vi "iTCread.vi"(0 "VISA resource name":refnum<visa-resource-name>, 1 "iTCreadCtrl":T1, 3 "error in (no error)":errorcluster) -> (7 "VISA resource name out":refnum<visa-resource-name>, 8 "number":dbl, 9 "read buffer":string, 10 "error out":errorcluster)   [LabVIEW 2017]
uses:
  controls/iTCreadCtrl.ctl
  <vilib>/regexp/Match Regular Expression.xnode
panel:
  out "read buffer 2":string
  out "after match":string
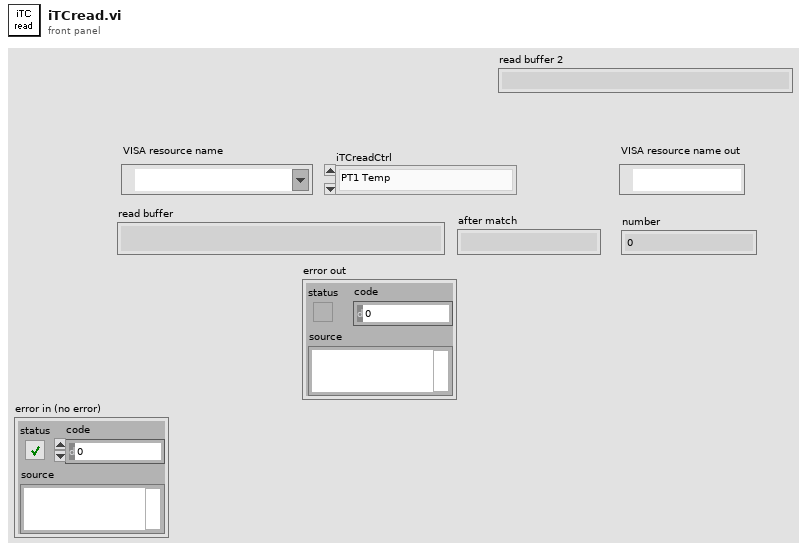
[diagram p1: front panel]
types:
  T1 = typedef "iTCreadCtrl.ctl" = enum16{"PT1 Temp", "PT2 Temp", "Sample Temp", "VTI Temp", "Needle Valve", "VTI Heater Power", "Sample Heater Power", "VTI Pressure"}
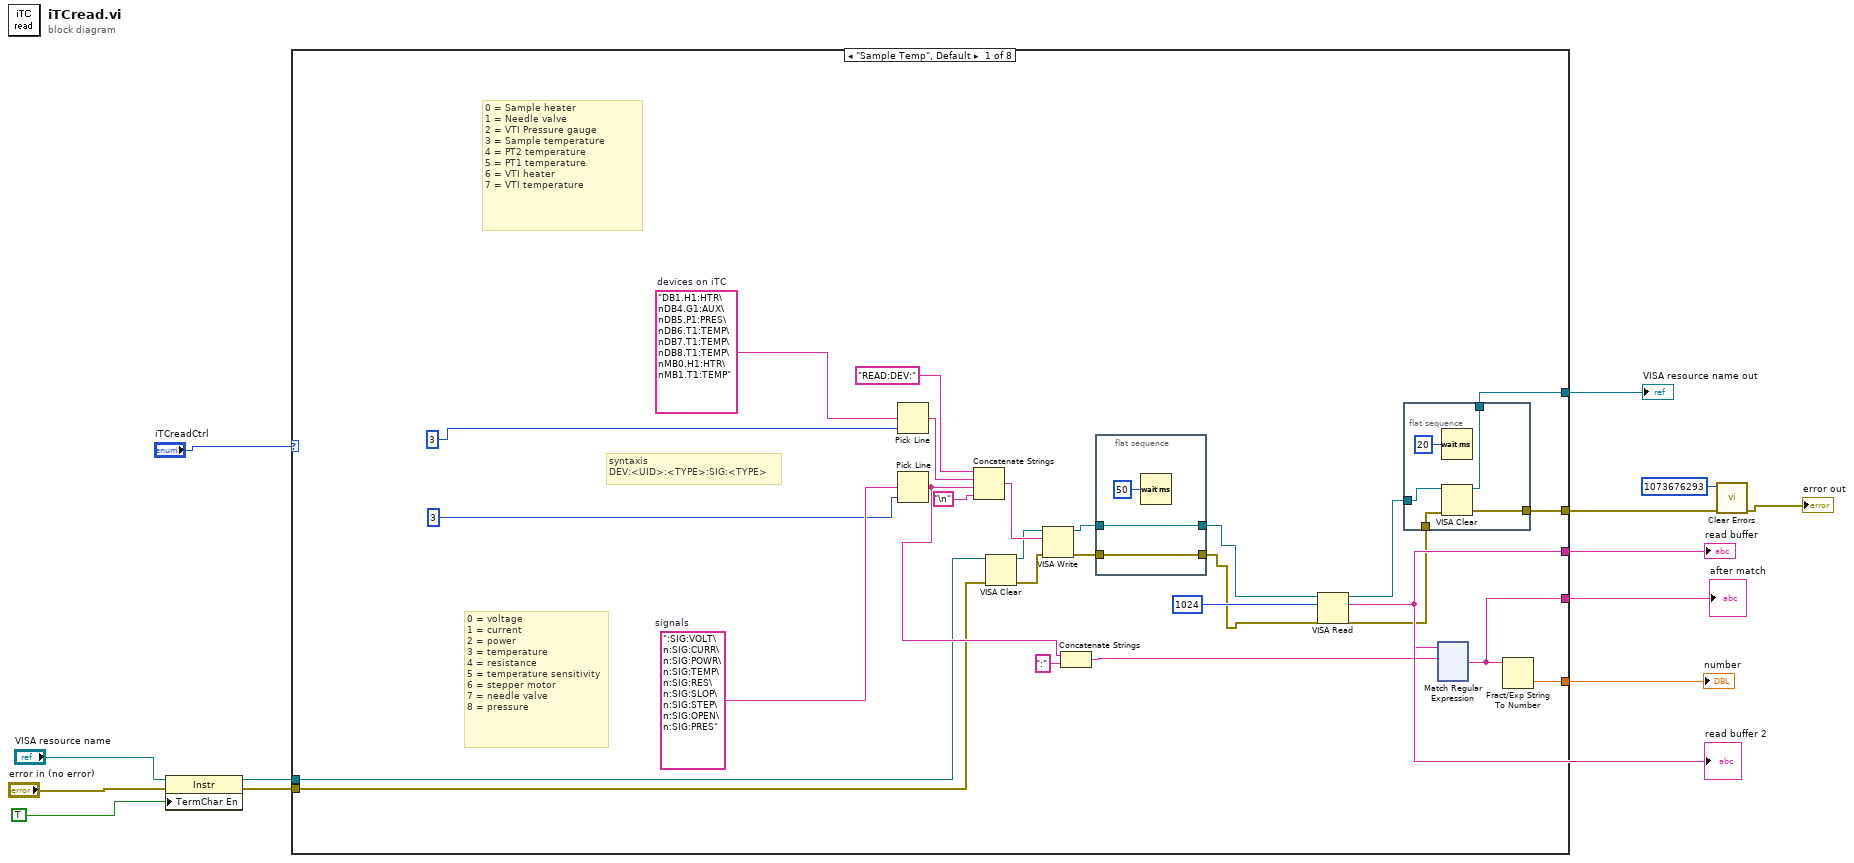
[diagram p0: block diagram]
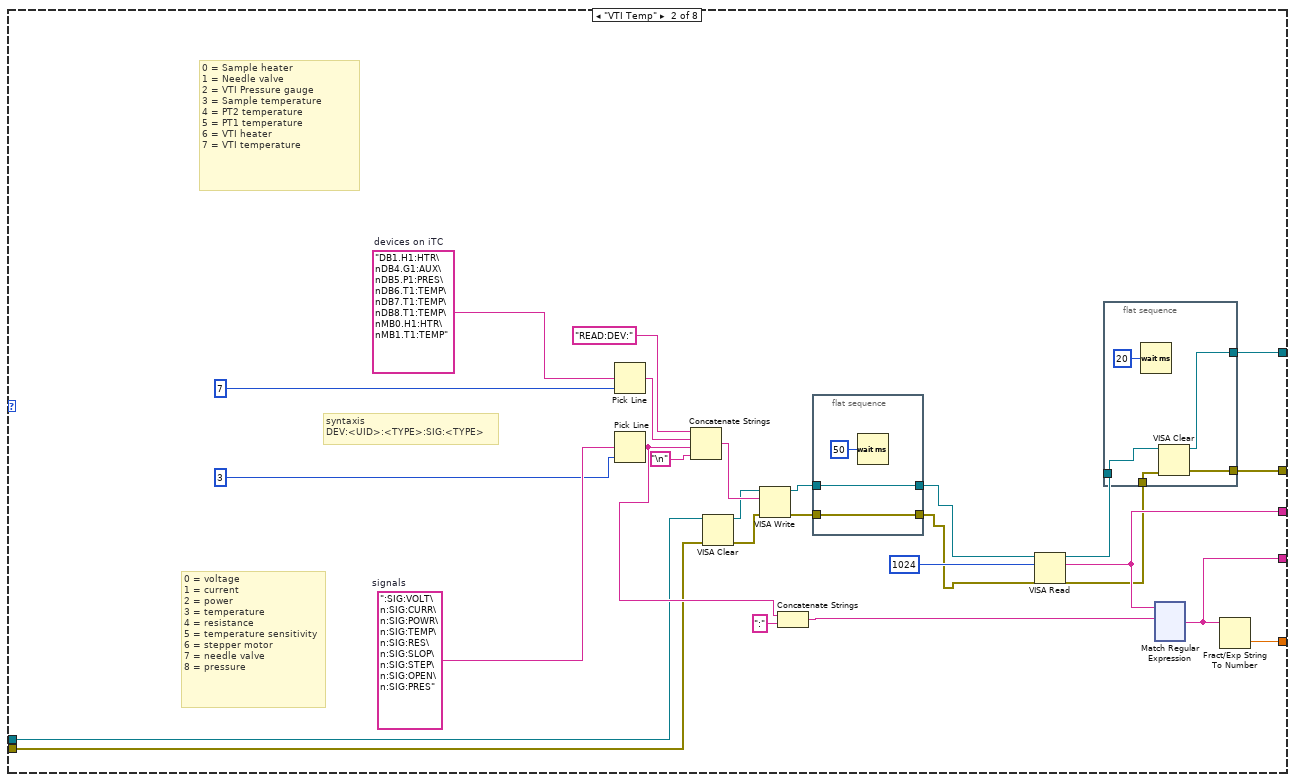
[diagram p2: hidden frame]
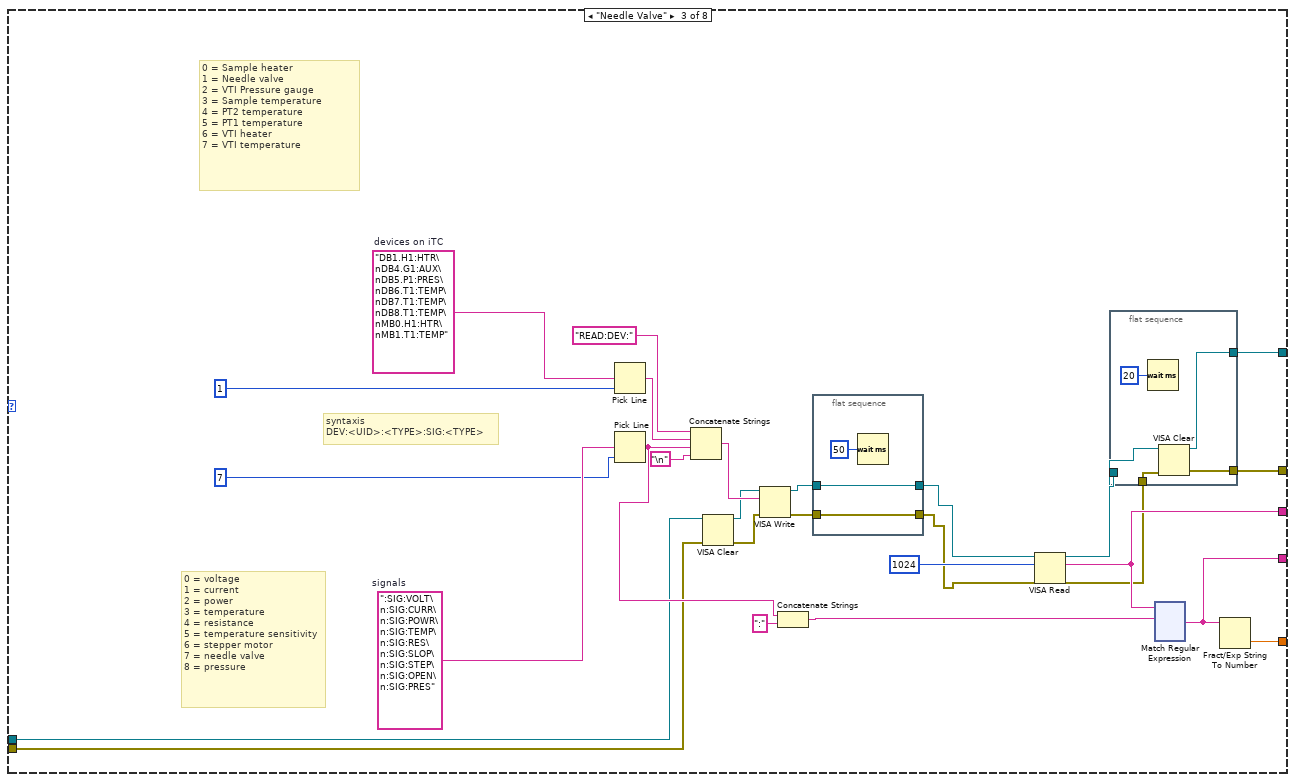
[diagram p3: hidden frame]
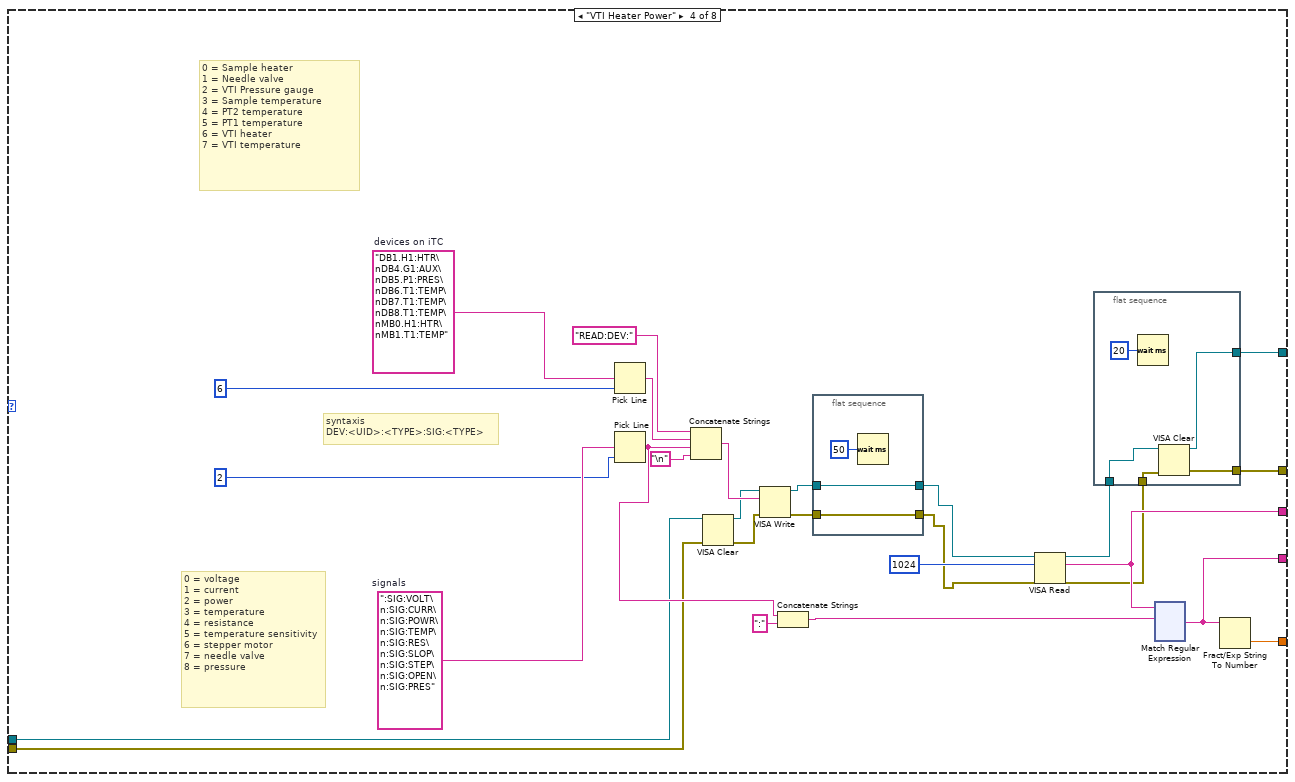
[diagram p4: hidden frame]
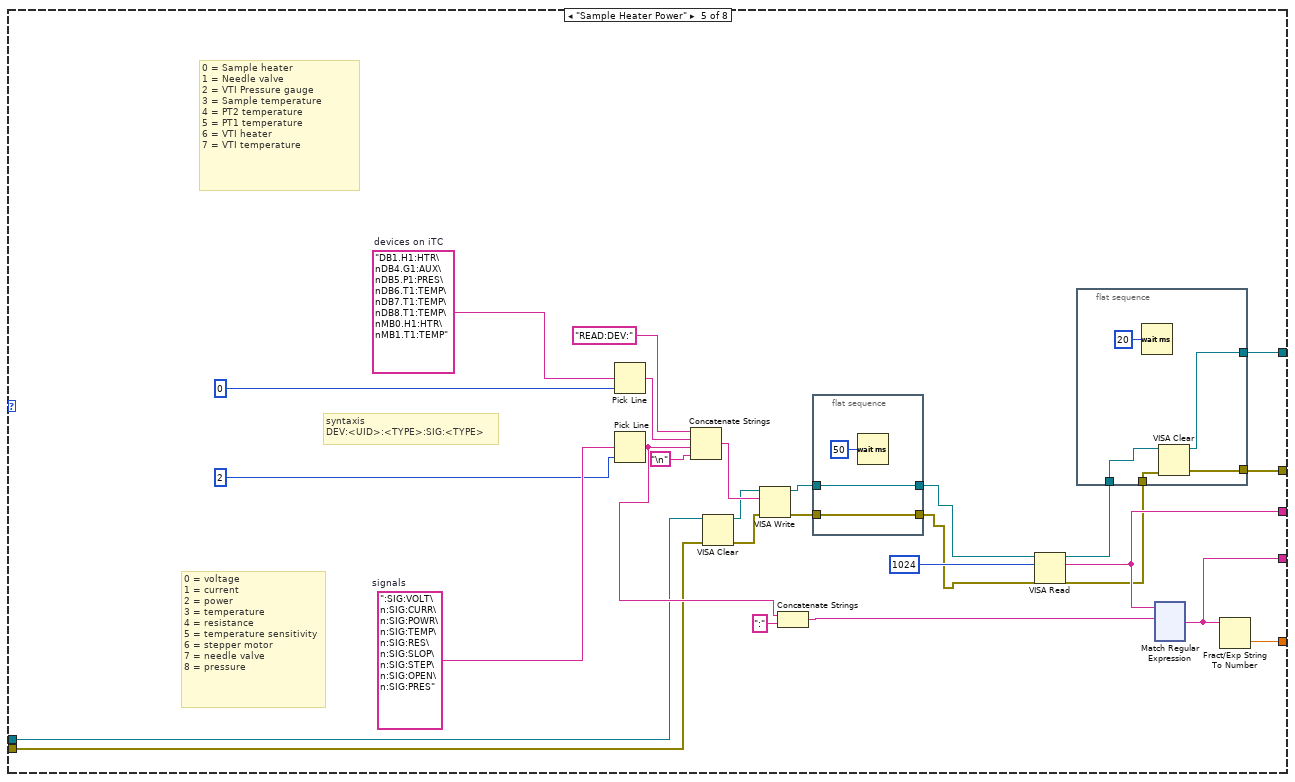
[diagram p5: hidden frame]
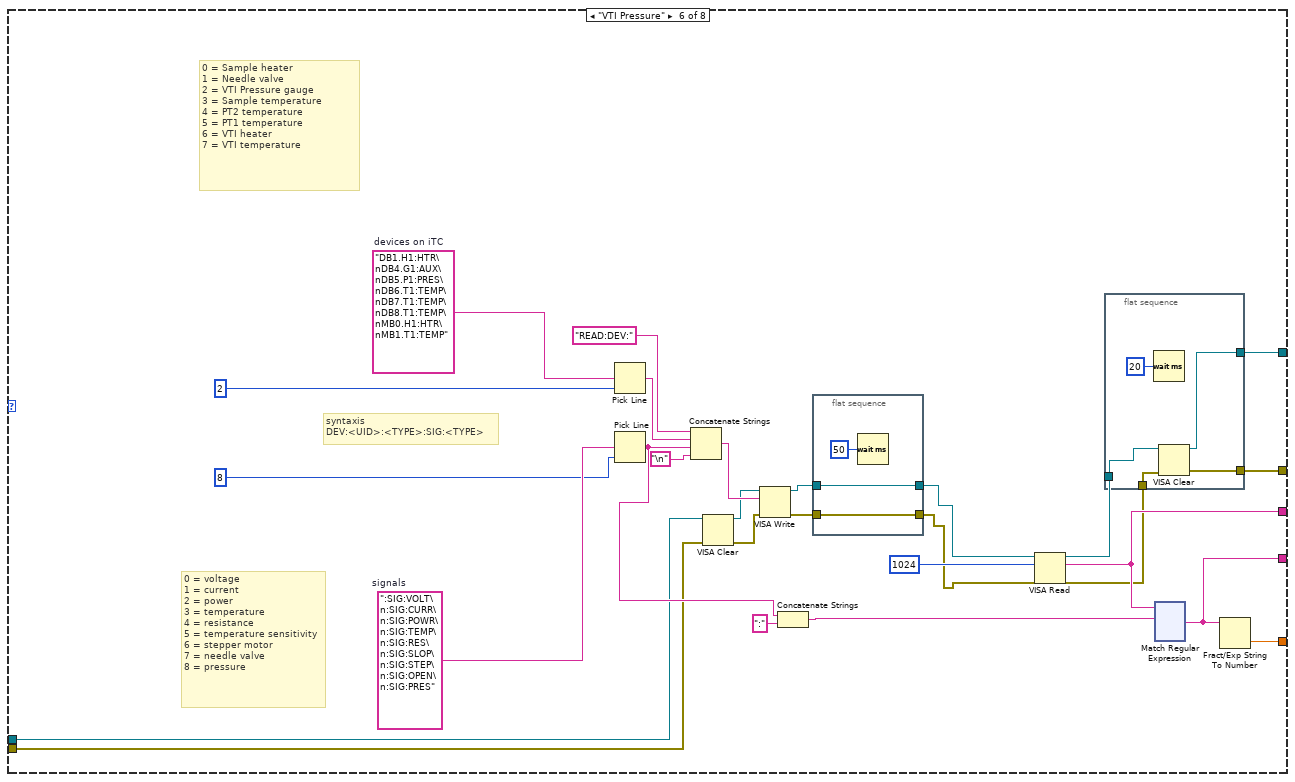
[diagram p6: hidden frame]
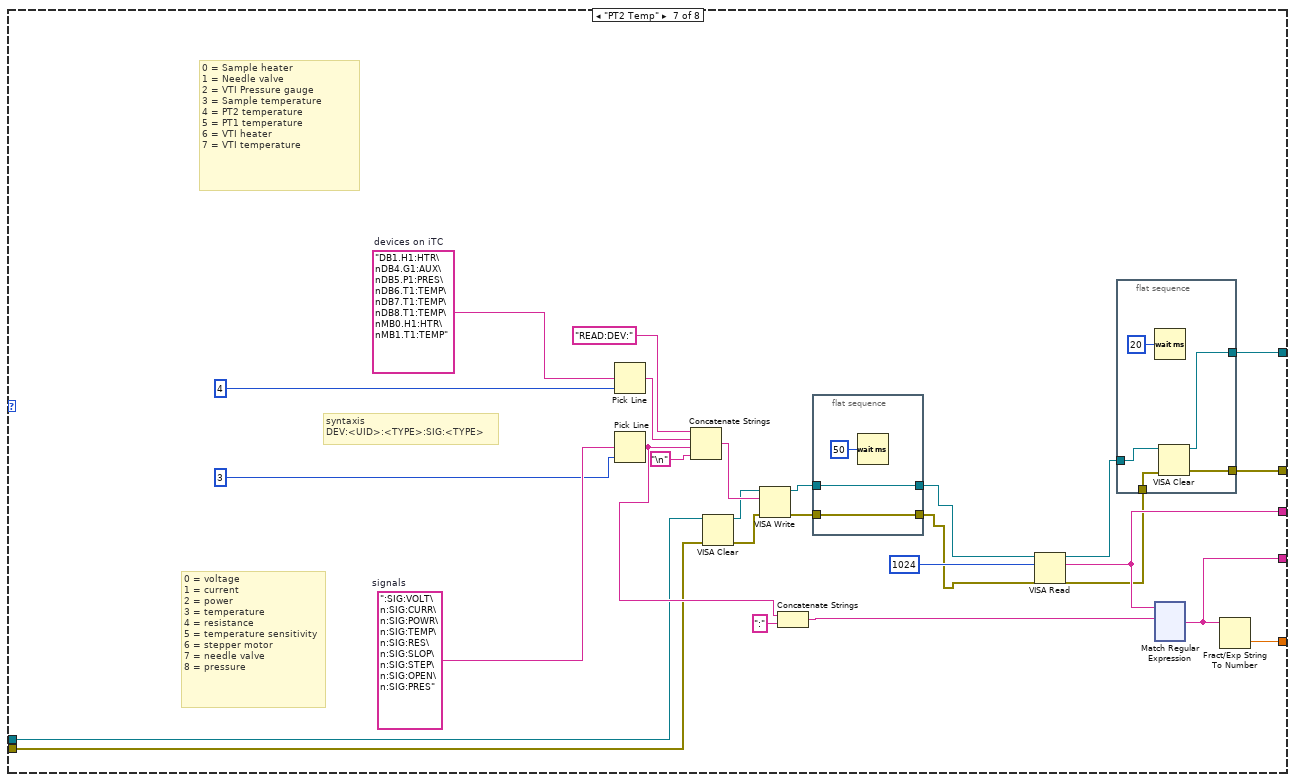
[diagram p7: hidden frame]
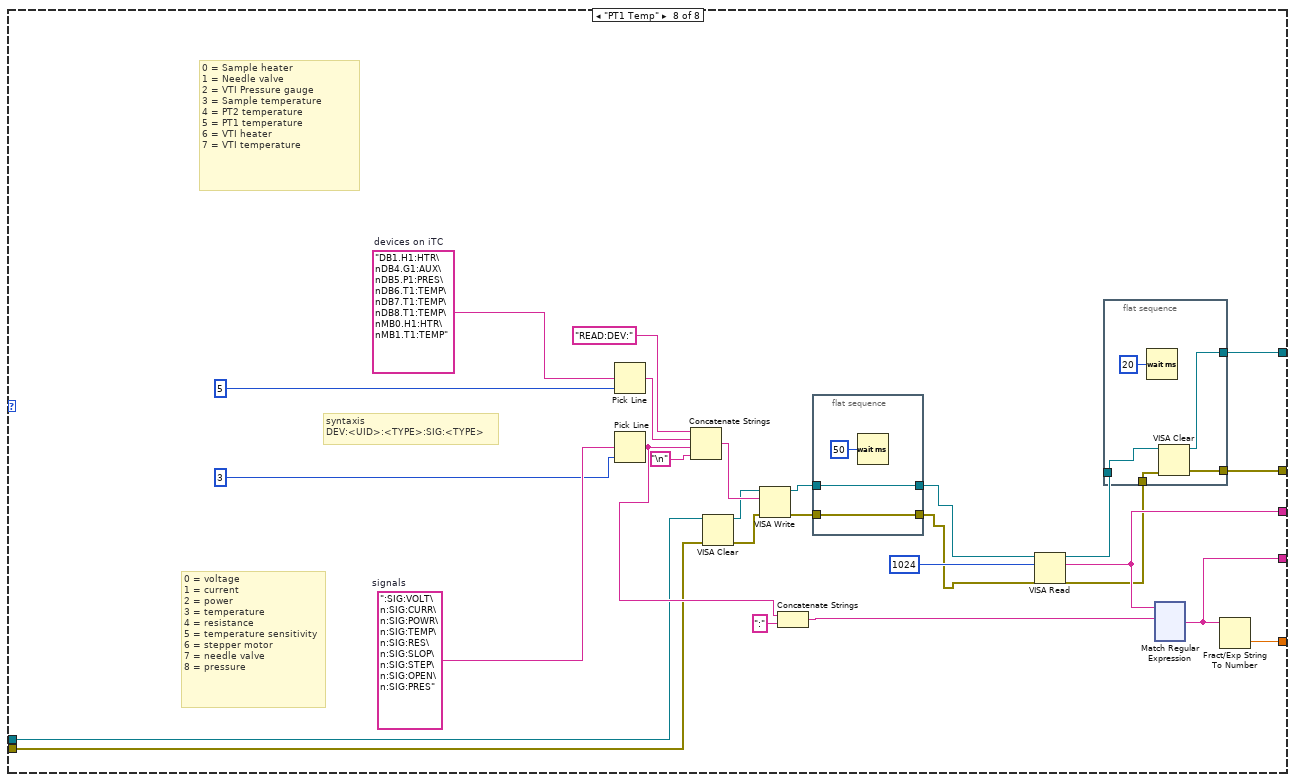
[diagram p8: hidden frame]
diagram:
  n1 = property class="Instr"(reference="VISA resource name", error in="error in (no error)", "TermChar En"=TRUE ("Message Based Settings:Termination Character Enable")) -> (reference out=w4:refnum<visa-resource-name>, error out=w5:errorcluster)
  n2 = case shown="\"Sample Temp\", Default" "iTCreadCtrl" {
    tunnel: [w40 w186 w332 w478 w624 w770 w916 w1062] -> w13
    tunnel: [w39 w185 w331 w477 w623 w769 w915 w1061] -> w12
    tunnel: [w38 w184 w330 w476 w622 w768 w914 w1060] -> w11
    tunnel: [w37 w183 w329 w475 w621 w767 w913 w1059] -> w10
    tunnel: [w36 w182 w328 w474 w620 w766 w912 w1058] -> w7
    tunnel: w5 -> [w19 w165 w311 w457 w603 w749 w895 w1041]
    tunnel: w4 -> [w18 w164 w310 w456 w602 w748 w894 w1040]
    frame "Sample Temp", Default {
      w32 = ":SIG:VOLT\n:SIG:CURR\n:SIG:POWR\n:SIG:TEMP\n:SIG:RES\n:SIG:SLOP\n:SIG:STEP\n:SIG:OPEN\n:SIG:PRES"  # signals
      w35 = "DB1.H1:HTR\nDB4.G1:AUX\nDB5.P1:PRES\nDB6.T1:TEMP\nDB7.T1:TEMP\nDB8.T1:TEMP\nMB0.H1:HTR\nMB1.T1:TEMP"  # devices on iTC
      # "0 = Sample heater\n1 = Needle valve\n2 = VTI Pressure gauge\n3 = Sample temperature\n4 = PT2 temperature\n5 = PT1 temperature\n6 = VTI heater\n7 = VTI temperature"
      # "0 = voltage\n1 = current\n2 = power\n3 = temperature\n4 = resistance\n5 = temperature sensitivity\n6 = stepper motor\n7 = needle valve\n8 = pressure"
      # "syntaxis\nDEV:<UID>:<TYPE>:SIG:<TYPE>"
      n3 = Pick Line(multi-line string=w35, line index=3) -> (output string=w33:string)  [unwired: 1 in]
      n4 = Pick Line(multi-line string=w32, line index=3) -> (output string=w29:string)  [unwired: 1 in]
      n5 = Concatenate Strings("READ:DEV:" ("write buffer"), w33, w29, "\n") -> (w31:string)
      n6 = VISA Clear(VISA resource name=w18, error in (no error)=w19) -> (VISA resource name out=w22:refnum<visa-resource-name>, error out=w23:errorcluster)
      n7 = VISA Write(VISA resource name=w22, write buffer=w31, error in (no error)=w23) -> (VISA resource name out=w17:refnum<visa-resource-name>, error out=w16:errorcluster)  [unwired: 1 out]
      n8 = Concatenate Strings(w29, ":" ("string")) -> (w28:string)
      n9 = flat-sequence {
        tunnel: w17 -> [w48]
        tunnel: w16 -> [w47]
        tunnel: [w48] -> w15
        tunnel: [w47] -> w14
        frame #0 {
          n10 = Wait (ms)(milliseconds to wait=u32 50) -> ()  [unwired: 1 out]
        }
      }
      n11 = VISA Read(VISA resource name=w15, byte count=u32 1024, error in (no error)=w14) -> (VISA resource name out=w21:refnum<visa-resource-name>, read buffer=w38:string, error out=w24:errorcluster)  [unwired: 1 out]
      n12 = flat-sequence {
        tunnel: [w45] -> w37
        tunnel: [w44] -> w36
        tunnel: w24 -> [w43]
        tunnel: w21 -> [w42]
        frame #0 {
          n13 = Wait (ms)(milliseconds to wait=u32 20) -> ()  [unwired: 1 out]
          n14 = VISA Clear(VISA resource name=w42, error in (no error)=w43) -> (VISA resource name out=w44:refnum<visa-resource-name>, error out=w45:errorcluster)
        }
      }
      n15 = xnode "Match Regular Expression"("input string"=w38, "regular expression"=w28) -> ("after match"=w40:string)  [unwired: 4 in, 4 out]
      n16 = Fract/Exp String To Number(string=w40) -> (number=w39:dbl)  [unwired: 3 in, 1 out]
    }
    frame "VTI Temp" {
      w178 = ":SIG:VOLT\n:SIG:CURR\n:SIG:POWR\n:SIG:TEMP\n:SIG:RES\n:SIG:SLOP\n:SIG:STEP\n:SIG:OPEN\n:SIG:PRES"  # signals
      w181 = "DB1.H1:HTR\nDB4.G1:AUX\nDB5.P1:PRES\nDB6.T1:TEMP\nDB7.T1:TEMP\nDB8.T1:TEMP\nMB0.H1:HTR\nMB1.T1:TEMP"  # devices on iTC
      # "0 = Sample heater\n1 = Needle valve\n2 = VTI Pressure gauge\n3 = Sample temperature\n4 = PT2 temperature\n5 = PT1 temperature\n6 = VTI heater\n7 = VTI temperature"
      # "0 = voltage\n1 = current\n2 = power\n3 = temperature\n4 = resistance\n5 = temperature sensitivity\n6 = stepper motor\n7 = needle valve\n8 = pressure"
      # "syntaxis\nDEV:<UID>:<TYPE>:SIG:<TYPE>"
      n17 = Pick Line(multi-line string=w181, line index=7) -> (output string=w179:string)  [unwired: 1 in]
      n18 = Pick Line(multi-line string=w178, line index=3) -> (output string=w175:string)  [unwired: 1 in]
      n19 = Concatenate Strings("READ:DEV:" ("write buffer"), w179, w175, "\n") -> (w177:string)
      n20 = VISA Clear(VISA resource name=w164, error in (no error)=w165) -> (VISA resource name out=w168:refnum<visa-resource-name>, error out=w169:errorcluster)
      n21 = VISA Write(VISA resource name=w168, write buffer=w177, error in (no error)=w169) -> (VISA resource name out=w163:refnum<visa-resource-name>, error out=w162:errorcluster)  [unwired: 1 out]
      n22 = Concatenate Strings(w175, ":" ("string")) -> (w174:string)
      n23 = flat-sequence {
        tunnel: w163 -> [w194]
        tunnel: w162 -> [w193]
        tunnel: [w194] -> w161
        tunnel: [w193] -> w160
        frame #0 {
          n24 = Wait (ms)(milliseconds to wait=u32 50) -> ()  [unwired: 1 out]
        }
      }
      n25 = VISA Read(VISA resource name=w161, byte count=u32 1024, error in (no error)=w160) -> (VISA resource name out=w167:refnum<visa-resource-name>, read buffer=w184:string, error out=w170:errorcluster)  [unwired: 1 out]
      n26 = flat-sequence {
        tunnel: [w191] -> w183
        tunnel: [w190] -> w182
        tunnel: w170 -> [w189]
        tunnel: w167 -> [w188]
        frame #0 {
          n27 = Wait (ms)(milliseconds to wait=u32 20) -> ()  [unwired: 1 out]
          n28 = VISA Clear(VISA resource name=w188, error in (no error)=w189) -> (VISA resource name out=w190:refnum<visa-resource-name>, error out=w191:errorcluster)
        }
      }
      n29 = xnode "Match Regular Expression"("input string"=w184, "regular expression"=w174) -> ("after match"=w186:string)  [unwired: 4 in, 4 out]
      n30 = Fract/Exp String To Number(string=w186) -> (number=w185:dbl)  [unwired: 3 in, 1 out]
    }
    frame "Needle Valve" {
      w324 = ":SIG:VOLT\n:SIG:CURR\n:SIG:POWR\n:SIG:TEMP\n:SIG:RES\n:SIG:SLOP\n:SIG:STEP\n:SIG:OPEN\n:SIG:PRES"  # signals
      w327 = "DB1.H1:HTR\nDB4.G1:AUX\nDB5.P1:PRES\nDB6.T1:TEMP\nDB7.T1:TEMP\nDB8.T1:TEMP\nMB0.H1:HTR\nMB1.T1:TEMP"  # devices on iTC
      # "0 = Sample heater\n1 = Needle valve\n2 = VTI Pressure gauge\n3 = Sample temperature\n4 = PT2 temperature\n5 = PT1 temperature\n6 = VTI heater\n7 = VTI temperature"
      # "0 = voltage\n1 = current\n2 = power\n3 = temperature\n4 = resistance\n5 = temperature sensitivity\n6 = stepper motor\n7 = needle valve\n8 = pressure"
      # "syntaxis\nDEV:<UID>:<TYPE>:SIG:<TYPE>"
      n31 = Pick Line(multi-line string=w327, line index=1) -> (output string=w325:string)  [unwired: 1 in]
      n32 = Pick Line(multi-line string=w324, line index=7) -> (output string=w321:string)  [unwired: 1 in]
      n33 = Concatenate Strings("READ:DEV:" ("write buffer"), w325, w321, "\n") -> (w323:string)
      n34 = VISA Clear(VISA resource name=w310, error in (no error)=w311) -> (VISA resource name out=w314:refnum<visa-resource-name>, error out=w315:errorcluster)
      n35 = VISA Write(VISA resource name=w314, write buffer=w323, error in (no error)=w315) -> (VISA resource name out=w309:refnum<visa-resource-name>, error out=w308:errorcluster)  [unwired: 1 out]
      n36 = Concatenate Strings(w321, ":" ("string")) -> (w320:string)
      n37 = flat-sequence {
        tunnel: w309 -> [w340]
        tunnel: w308 -> [w339]
        tunnel: [w340] -> w307
        tunnel: [w339] -> w306
        frame #0 {
          n38 = Wait (ms)(milliseconds to wait=u32 50) -> ()  [unwired: 1 out]
        }
      }
      n39 = VISA Read(VISA resource name=w307, byte count=u32 1024, error in (no error)=w306) -> (VISA resource name out=w313:refnum<visa-resource-name>, read buffer=w330:string, error out=w316:errorcluster)  [unwired: 1 out]
      n40 = flat-sequence {
        tunnel: [w337] -> w329
        tunnel: [w336] -> w328
        tunnel: w316 -> [w335]
        tunnel: w313 -> [w334]
        frame #0 {
          n41 = Wait (ms)(milliseconds to wait=u32 20) -> ()  [unwired: 1 out]
          n42 = VISA Clear(VISA resource name=w334, error in (no error)=w335) -> (VISA resource name out=w336:refnum<visa-resource-name>, error out=w337:errorcluster)
        }
      }
      n43 = xnode "Match Regular Expression"("input string"=w330, "regular expression"=w320) -> ("after match"=w332:string)  [unwired: 4 in, 4 out]
      n44 = Fract/Exp String To Number(string=w332) -> (number=w331:dbl)  [unwired: 3 in, 1 out]
    }
    frame "VTI Heater Power" {
      w470 = ":SIG:VOLT\n:SIG:CURR\n:SIG:POWR\n:SIG:TEMP\n:SIG:RES\n:SIG:SLOP\n:SIG:STEP\n:SIG:OPEN\n:SIG:PRES"  # signals
      w473 = "DB1.H1:HTR\nDB4.G1:AUX\nDB5.P1:PRES\nDB6.T1:TEMP\nDB7.T1:TEMP\nDB8.T1:TEMP\nMB0.H1:HTR\nMB1.T1:TEMP"  # devices on iTC
      # "0 = Sample heater\n1 = Needle valve\n2 = VTI Pressure gauge\n3 = Sample temperature\n4 = PT2 temperature\n5 = PT1 temperature\n6 = VTI heater\n7 = VTI temperature"
      # "0 = voltage\n1 = current\n2 = power\n3 = temperature\n4 = resistance\n5 = temperature sensitivity\n6 = stepper motor\n7 = needle valve\n8 = pressure"
      # "syntaxis\nDEV:<UID>:<TYPE>:SIG:<TYPE>"
      n45 = Pick Line(multi-line string=w473, line index=6) -> (output string=w471:string)  [unwired: 1 in]
      n46 = Pick Line(multi-line string=w470, line index=2) -> (output string=w467:string)  [unwired: 1 in]
      n47 = Concatenate Strings("READ:DEV:" ("write buffer"), w471, w467, "\n") -> (w469:string)
      n48 = VISA Clear(VISA resource name=w456, error in (no error)=w457) -> (VISA resource name out=w460:refnum<visa-resource-name>, error out=w461:errorcluster)
      n49 = VISA Write(VISA resource name=w460, write buffer=w469, error in (no error)=w461) -> (VISA resource name out=w455:refnum<visa-resource-name>, error out=w454:errorcluster)  [unwired: 1 out]
      n50 = Concatenate Strings(w467, ":" ("string")) -> (w466:string)
      n51 = flat-sequence {
        tunnel: w455 -> [w486]
        tunnel: w454 -> [w485]
        tunnel: [w486] -> w453
        tunnel: [w485] -> w452
        frame #0 {
          n52 = Wait (ms)(milliseconds to wait=u32 50) -> ()  [unwired: 1 out]
        }
      }
      n53 = VISA Read(VISA resource name=w453, byte count=u32 1024, error in (no error)=w452) -> (VISA resource name out=w459:refnum<visa-resource-name>, read buffer=w476:string, error out=w462:errorcluster)  [unwired: 1 out]
      n54 = flat-sequence {
        tunnel: [w483] -> w475
        tunnel: [w482] -> w474
        tunnel: w462 -> [w481]
        tunnel: w459 -> [w480]
        frame #0 {
          n55 = Wait (ms)(milliseconds to wait=u32 20) -> ()  [unwired: 1 out]
          n56 = VISA Clear(VISA resource name=w480, error in (no error)=w481) -> (VISA resource name out=w482:refnum<visa-resource-name>, error out=w483:errorcluster)
        }
      }
      n57 = xnode "Match Regular Expression"("input string"=w476, "regular expression"=w466) -> ("after match"=w478:string)  [unwired: 4 in, 4 out]
      n58 = Fract/Exp String To Number(string=w478) -> (number=w477:dbl)  [unwired: 3 in, 1 out]
    }
    frame "Sample Heater Power" {
      w616 = ":SIG:VOLT\n:SIG:CURR\n:SIG:POWR\n:SIG:TEMP\n:SIG:RES\n:SIG:SLOP\n:SIG:STEP\n:SIG:OPEN\n:SIG:PRES"  # signals
      w619 = "DB1.H1:HTR\nDB4.G1:AUX\nDB5.P1:PRES\nDB6.T1:TEMP\nDB7.T1:TEMP\nDB8.T1:TEMP\nMB0.H1:HTR\nMB1.T1:TEMP"  # devices on iTC
      # "0 = Sample heater\n1 = Needle valve\n2 = VTI Pressure gauge\n3 = Sample temperature\n4 = PT2 temperature\n5 = PT1 temperature\n6 = VTI heater\n7 = VTI temperature"
      # "0 = voltage\n1 = current\n2 = power\n3 = temperature\n4 = resistance\n5 = temperature sensitivity\n6 = stepper motor\n7 = needle valve\n8 = pressure"
      # "syntaxis\nDEV:<UID>:<TYPE>:SIG:<TYPE>"
      n59 = Pick Line(multi-line string=w619, line index=0) -> (output string=w617:string)  [unwired: 1 in]
      n60 = Pick Line(multi-line string=w616, line index=2) -> (output string=w613:string)  [unwired: 1 in]
      n61 = Concatenate Strings("READ:DEV:" ("write buffer"), w617, w613, "\n") -> (w615:string)
      n62 = VISA Clear(VISA resource name=w602, error in (no error)=w603) -> (VISA resource name out=w606:refnum<visa-resource-name>, error out=w607:errorcluster)
      n63 = VISA Write(VISA resource name=w606, write buffer=w615, error in (no error)=w607) -> (VISA resource name out=w601:refnum<visa-resource-name>, error out=w600:errorcluster)  [unwired: 1 out]
      n64 = Concatenate Strings(w613, ":" ("string")) -> (w612:string)
      n65 = flat-sequence {
        tunnel: w601 -> [w632]
        tunnel: w600 -> [w631]
        tunnel: [w632] -> w599
        tunnel: [w631] -> w598
        frame #0 {
          n66 = Wait (ms)(milliseconds to wait=u32 50) -> ()  [unwired: 1 out]
        }
      }
      n67 = VISA Read(VISA resource name=w599, byte count=u32 1024, error in (no error)=w598) -> (VISA resource name out=w605:refnum<visa-resource-name>, read buffer=w622:string, error out=w608:errorcluster)  [unwired: 1 out]
      n68 = flat-sequence {
        tunnel: [w629] -> w621
        tunnel: [w628] -> w620
        tunnel: w608 -> [w627]
        tunnel: w605 -> [w626]
        frame #0 {
          n69 = Wait (ms)(milliseconds to wait=u32 20) -> ()  [unwired: 1 out]
          n70 = VISA Clear(VISA resource name=w626, error in (no error)=w627) -> (VISA resource name out=w628:refnum<visa-resource-name>, error out=w629:errorcluster)
        }
      }
      n71 = xnode "Match Regular Expression"("input string"=w622, "regular expression"=w612) -> ("after match"=w624:string)  [unwired: 4 in, 4 out]
      n72 = Fract/Exp String To Number(string=w624) -> (number=w623:dbl)  [unwired: 3 in, 1 out]
    }
    frame "VTI Pressure" {
      w762 = ":SIG:VOLT\n:SIG:CURR\n:SIG:POWR\n:SIG:TEMP\n:SIG:RES\n:SIG:SLOP\n:SIG:STEP\n:SIG:OPEN\n:SIG:PRES"  # signals
      w765 = "DB1.H1:HTR\nDB4.G1:AUX\nDB5.P1:PRES\nDB6.T1:TEMP\nDB7.T1:TEMP\nDB8.T1:TEMP\nMB0.H1:HTR\nMB1.T1:TEMP"  # devices on iTC
      # "0 = Sample heater\n1 = Needle valve\n2 = VTI Pressure gauge\n3 = Sample temperature\n4 = PT2 temperature\n5 = PT1 temperature\n6 = VTI heater\n7 = VTI temperature"
      # "0 = voltage\n1 = current\n2 = power\n3 = temperature\n4 = resistance\n5 = temperature sensitivity\n6 = stepper motor\n7 = needle valve\n8 = pressure"
      # "syntaxis\nDEV:<UID>:<TYPE>:SIG:<TYPE>"
      n73 = Pick Line(multi-line string=w765, line index=2) -> (output string=w763:string)  [unwired: 1 in]
      n74 = Pick Line(multi-line string=w762, line index=8) -> (output string=w759:string)  [unwired: 1 in]
      n75 = Concatenate Strings("READ:DEV:" ("write buffer"), w763, w759, "\n") -> (w761:string)
      n76 = VISA Clear(VISA resource name=w748, error in (no error)=w749) -> (VISA resource name out=w752:refnum<visa-resource-name>, error out=w753:errorcluster)
      n77 = VISA Write(VISA resource name=w752, write buffer=w761, error in (no error)=w753) -> (VISA resource name out=w747:refnum<visa-resource-name>, error out=w746:errorcluster)  [unwired: 1 out]
      n78 = Concatenate Strings(w759, ":" ("string")) -> (w758:string)
      n79 = flat-sequence {
        tunnel: w747 -> [w778]
        tunnel: w746 -> [w777]
        tunnel: [w778] -> w745
        tunnel: [w777] -> w744
        frame #0 {
          n80 = Wait (ms)(milliseconds to wait=u32 50) -> ()  [unwired: 1 out]
        }
      }
      n81 = VISA Read(VISA resource name=w745, byte count=u32 1024, error in (no error)=w744) -> (VISA resource name out=w751:refnum<visa-resource-name>, read buffer=w768:string, error out=w754:errorcluster)  [unwired: 1 out]
      n82 = flat-sequence {
        tunnel: [w775] -> w767
        tunnel: [w774] -> w766
        tunnel: w754 -> [w773]
        tunnel: w751 -> [w772]
        frame #0 {
          n83 = Wait (ms)(milliseconds to wait=u32 20) -> ()  [unwired: 1 out]
          n84 = VISA Clear(VISA resource name=w772, error in (no error)=w773) -> (VISA resource name out=w774:refnum<visa-resource-name>, error out=w775:errorcluster)
        }
      }
      n85 = xnode "Match Regular Expression"("input string"=w768, "regular expression"=w758) -> ("after match"=w770:string)  [unwired: 4 in, 4 out]
      n86 = Fract/Exp String To Number(string=w770) -> (number=w769:dbl)  [unwired: 3 in, 1 out]
    }
    frame "PT2 Temp" {
      w908 = ":SIG:VOLT\n:SIG:CURR\n:SIG:POWR\n:SIG:TEMP\n:SIG:RES\n:SIG:SLOP\n:SIG:STEP\n:SIG:OPEN\n:SIG:PRES"  # signals
      w911 = "DB1.H1:HTR\nDB4.G1:AUX\nDB5.P1:PRES\nDB6.T1:TEMP\nDB7.T1:TEMP\nDB8.T1:TEMP\nMB0.H1:HTR\nMB1.T1:TEMP"  # devices on iTC
      # "0 = Sample heater\n1 = Needle valve\n2 = VTI Pressure gauge\n3 = Sample temperature\n4 = PT2 temperature\n5 = PT1 temperature\n6 = VTI heater\n7 = VTI temperature"
      # "0 = voltage\n1 = current\n2 = power\n3 = temperature\n4 = resistance\n5 = temperature sensitivity\n6 = stepper motor\n7 = needle valve\n8 = pressure"
      # "syntaxis\nDEV:<UID>:<TYPE>:SIG:<TYPE>"
      n87 = Pick Line(multi-line string=w911, line index=4) -> (output string=w909:string)  [unwired: 1 in]
      n88 = Pick Line(multi-line string=w908, line index=3) -> (output string=w905:string)  [unwired: 1 in]
      n89 = Concatenate Strings("READ:DEV:" ("write buffer"), w909, w905, "\n") -> (w907:string)
      n90 = VISA Clear(VISA resource name=w894, error in (no error)=w895) -> (VISA resource name out=w898:refnum<visa-resource-name>, error out=w899:errorcluster)
      n91 = VISA Write(VISA resource name=w898, write buffer=w907, error in (no error)=w899) -> (VISA resource name out=w893:refnum<visa-resource-name>, error out=w892:errorcluster)  [unwired: 1 out]
      n92 = Concatenate Strings(w905, ":" ("string")) -> (w904:string)
      n93 = flat-sequence {
        tunnel: w893 -> [w924]
        tunnel: w892 -> [w923]
        tunnel: [w924] -> w891
        tunnel: [w923] -> w890
        frame #0 {
          n94 = Wait (ms)(milliseconds to wait=u32 50) -> ()  [unwired: 1 out]
        }
      }
      n95 = VISA Read(VISA resource name=w891, byte count=u32 1024, error in (no error)=w890) -> (VISA resource name out=w897:refnum<visa-resource-name>, read buffer=w914:string, error out=w900:errorcluster)  [unwired: 1 out]
      n96 = flat-sequence {
        tunnel: [w921] -> w913
        tunnel: [w920] -> w912
        tunnel: w900 -> [w919]
        tunnel: w897 -> [w918]
        frame #0 {
          n97 = Wait (ms)(milliseconds to wait=u32 20) -> ()  [unwired: 1 out]
          n98 = VISA Clear(VISA resource name=w918, error in (no error)=w919) -> (VISA resource name out=w920:refnum<visa-resource-name>, error out=w921:errorcluster)
        }
      }
      n99 = xnode "Match Regular Expression"("input string"=w914, "regular expression"=w904) -> ("after match"=w916:string)  [unwired: 4 in, 4 out]
      n100 = Fract/Exp String To Number(string=w916) -> (number=w915:dbl)  [unwired: 3 in, 1 out]
    }
    frame "PT1 Temp" {
      w1054 = ":SIG:VOLT\n:SIG:CURR\n:SIG:POWR\n:SIG:TEMP\n:SIG:RES\n:SIG:SLOP\n:SIG:STEP\n:SIG:OPEN\n:SIG:PRES"  # signals
      w1057 = "DB1.H1:HTR\nDB4.G1:AUX\nDB5.P1:PRES\nDB6.T1:TEMP\nDB7.T1:TEMP\nDB8.T1:TEMP\nMB0.H1:HTR\nMB1.T1:TEMP"  # devices on iTC
      # "0 = Sample heater\n1 = Needle valve\n2 = VTI Pressure gauge\n3 = Sample temperature\n4 = PT2 temperature\n5 = PT1 temperature\n6 = VTI heater\n7 = VTI temperature"
      # "0 = voltage\n1 = current\n2 = power\n3 = temperature\n4 = resistance\n5 = temperature sensitivity\n6 = stepper motor\n7 = needle valve\n8 = pressure"
      # "syntaxis\nDEV:<UID>:<TYPE>:SIG:<TYPE>"
      n101 = Pick Line(multi-line string=w1057, line index=5) -> (output string=w1055:string)  [unwired: 1 in]
      n102 = Pick Line(multi-line string=w1054, line index=3) -> (output string=w1051:string)  [unwired: 1 in]
      n103 = Concatenate Strings("READ:DEV:" ("write buffer"), w1055, w1051, "\n") -> (w1053:string)
      n104 = VISA Clear(VISA resource name=w1040, error in (no error)=w1041) -> (VISA resource name out=w1044:refnum<visa-resource-name>, error out=w1045:errorcluster)
      n105 = VISA Write(VISA resource name=w1044, write buffer=w1053, error in (no error)=w1045) -> (VISA resource name out=w1039:refnum<visa-resource-name>, error out=w1038:errorcluster)  [unwired: 1 out]
      n106 = Concatenate Strings(w1051, ":" ("string")) -> (w1050:string)
      n107 = flat-sequence {
        tunnel: w1039 -> [w1070]
        tunnel: w1038 -> [w1069]
        tunnel: [w1070] -> w1037
        tunnel: [w1069] -> w1036
        frame #0 {
          n108 = Wait (ms)(milliseconds to wait=u32 50) -> ()  [unwired: 1 out]
        }
      }
      n109 = VISA Read(VISA resource name=w1037, byte count=u32 1024, error in (no error)=w1036) -> (VISA resource name out=w1043:refnum<visa-resource-name>, read buffer=w1060:string, error out=w1046:errorcluster)  [unwired: 1 out]
      n110 = flat-sequence {
        tunnel: [w1067] -> w1059
        tunnel: [w1066] -> w1058
        tunnel: w1046 -> [w1065]
        tunnel: w1043 -> [w1064]
        frame #0 {
          n111 = Wait (ms)(milliseconds to wait=u32 20) -> ()  [unwired: 1 out]
          n112 = VISA Clear(VISA resource name=w1064, error in (no error)=w1065) -> (VISA resource name out=w1066:refnum<visa-resource-name>, error out=w1067:errorcluster)
        }
      }
      n113 = xnode "Match Regular Expression"("input string"=w1060, "regular expression"=w1050) -> ("after match"=w1062:string)  [unwired: 4 in, 4 out]
      n114 = Fract/Exp String To Number(string=w1062) -> (number=w1061:dbl)  [unwired: 3 in, 1 out]
    }
  }
  "read buffer" <- w11
  "VISA resource name out" <- w7
  "after match" <- w13
  "number" <- w12
  "read buffer 2" <- w11
  n115 = call <vilib>:"Clear Errors.vi"("error in (no error)"=w10, "specific error code to clear (0: all)"=1073676293) -> ("error out"=→"error out":errorcluster)  [unwired: 4 in, 1 out]
